vi "flatten.vi"(8 "error in (no error)":errorcluster, 11 "PID Loop in":refnum<class "PID Loop.lvclass">) -> (0 "error out":errorcluster, 3 "flattened PID Loop":string)   [LabVIEW 2014, in "PID Loop.lvclass"]
uses:
  PID Loop.lvclass
  PID Loop.lvclass/PID Loop.ctl
  <vilib>/NI/Configuration Framework/serializable configuration/NISE_CEF_serializable configuration.lvclass
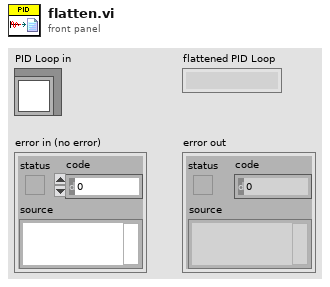
[diagram p1: front panel]
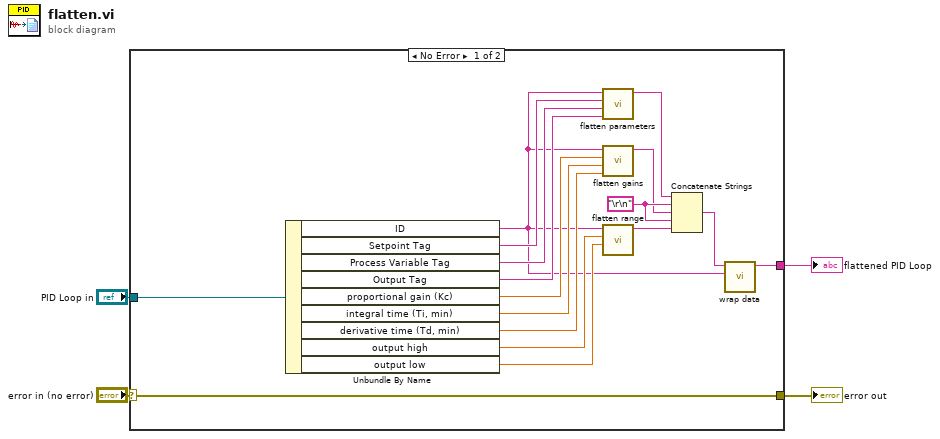
[diagram p0: block diagram]
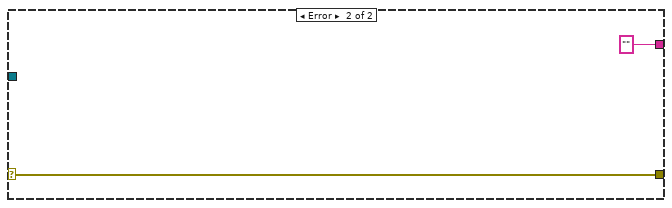
[diagram p2: hidden frame]
diagram:
  n1 = case shown="No Error" "error in (no error)" {
    selector: "error in (no error)" -> [w21 w23]
    tunnel: [w21 w23] -> w3
    tunnel: "PID Loop in" -> [w5 _]
    tunnel: [w6 "" ("wrapped data")] -> w1
    frame No Error {
      w11 = "\r\n"
      n2 = Unbundle By Name(w5) -> ("ID"=w12:string, "Setpoint Tag"=w16:string, "Process Variable Tag"=w15:string, "Output Tag"=w14:string, "proportional gain (Kc)"=w18:dbl, "integral time (Ti, min)"=w17:dbl, "derivative time (Td, min)"=w13:dbl, "output high"=w19:dbl, "output low"=w20:dbl)
      n3 = call "flatten parameters.vi"("Output Tag"=w14, "Process Variable Tag"=w15, "Setpoint Tag"=w16, "ID"=w12) -> ("wrapped data"=w10:string)  [unwired: 7 in]
      n4 = call "flatten gains.vi"("derivative time (Td, min)"=w13, "integral time (Ti, min)"=w17, "proportional gain (Kc)"=w18, "ID"=w12) -> ("wrapped data"=w9:string)  [unwired: 7 in]
      n5 = call "flatten range.vi"("output low"=w20, "output high"=w19, "ID"=w12) -> ("wrapped data"=w8:string)  [unwired: 8 in]
      n6 = Concatenate Strings(w10, w11, w9, w11, w8) -> (w7:string)
      n7 = call <vilib>:"wrap data.vi"("identifier"=w12, "data to wrap"=w7) -> ("wrapped data"=w6:string)  [unwired: 9 in]
    }
    frame Error {
    }
  }
  "error out" <- w3
  "flattened PID Loop" <- w1
